vi "датчик.vi"() -> ()   [LabVIEW 2019]
panel:
  in  "Boolean":bool
  out "Numeric":dbl
  in  "stop":bool
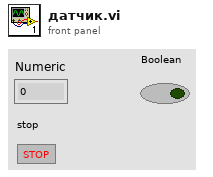
[diagram p1: front panel]
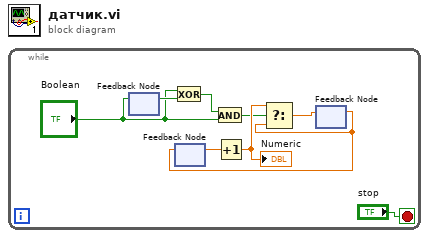
[diagram p0: block diagram]
diagram:
  n1 = while {
    stop <- "stop" stop-if-true
    n2 = feedback #1() -> (w5:bool)  [unwired: 1 in]
    n3 = feedback-in #1("Boolean") -> ()
    n4 = Exclusive Or(1:w5, 2:"Boolean") -> (0:w4:bool)
    n5 = feedback #2() -> (w9:dbl)  [unwired: 1 in]
    n6 = And(x=w4, y="Boolean") -> (x .and. y?=w3:bool)
    n7 = Increment(x=w9) -> (x+1=w8:dbl)
    "Numeric" <- w8
    n8 = feedback #3() -> (w6:dbl)  [unwired: 1 in]
    n9 = feedback-in #2(w6) -> ()
    n10 = Select(t=w8, s=w3, f=w6) -> (s? t:f=w7:dbl)
    n11 = feedback-in #3(w7) -> ()
  }
